vi "sv_Check for AvgParam Change [Octave].vi"(6 "averaging type":T2(ring), 7 "restart averaging (F) /reset":bool, 8 "error in (no error)":errorcluster, 9 "equal confidence level [dB]":dbl=1.0 format="%.2f", 10 "exp avg settings":T1={" mode"=enum."Fast", "time constant [ms]"=125.0} {"time constant [ms]" format="%.2f"}) -> (0 "error out":errorcluster, 2 "Param_has_changed":bool)   [LabVIEW 2017, in "SoundVib_Octave_2014 standard.lvlib"]
uses:
  <vilib>/addons/Sound and Vibration/svt_Octave/SoundVib_Octave_2014 standard.lvlib
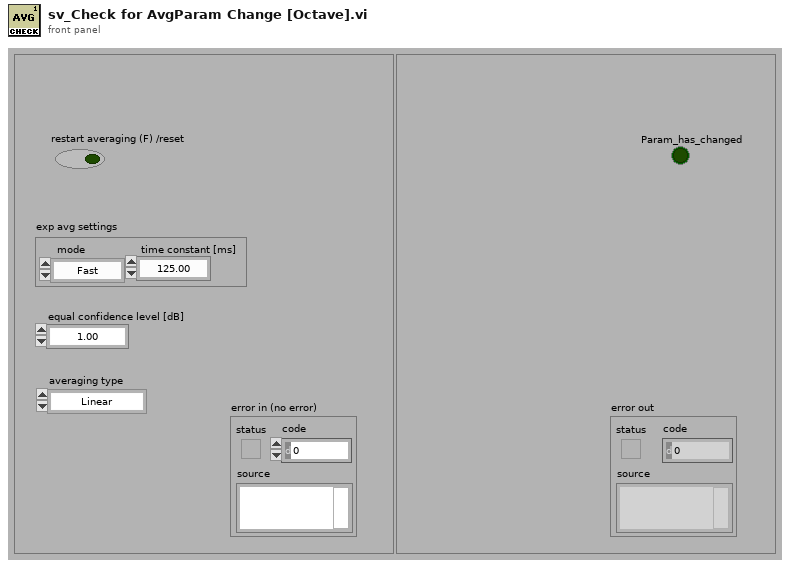
[diagram p1: front panel]
types:
  T1 = cluster{" mode":enum16{"Slow", "Fast", "Impulse", "Custom"}, "time constant [ms]":dbl}
  T2 = enum16{"Linear", "Exponential", "Equal confidence", "Peak"}
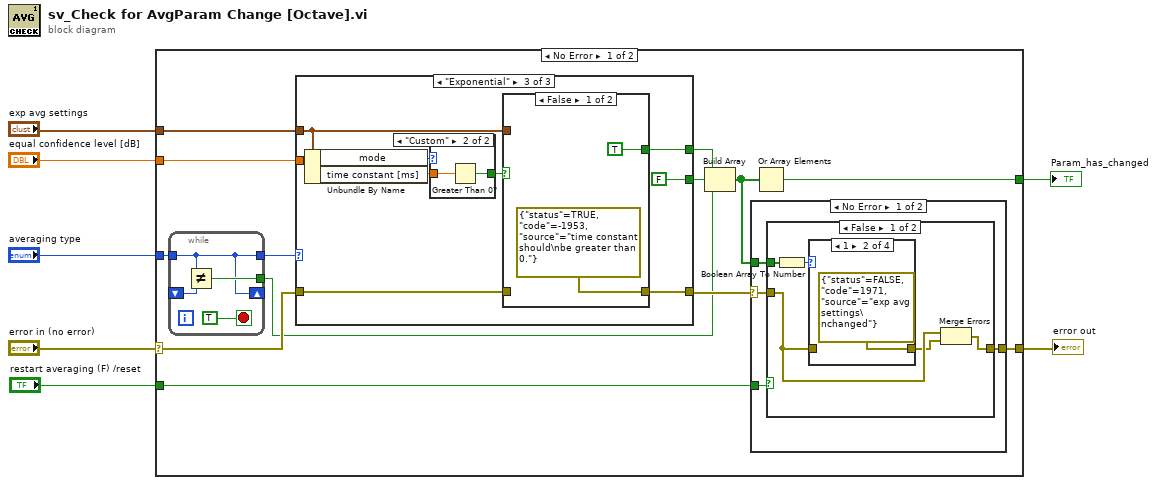
[diagram p0: block diagram]
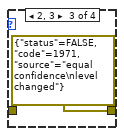
[diagram p3: hidden frame]
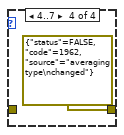
[diagram p4: hidden frame]
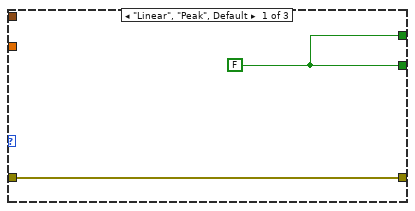
[diagram p7: hidden frame]
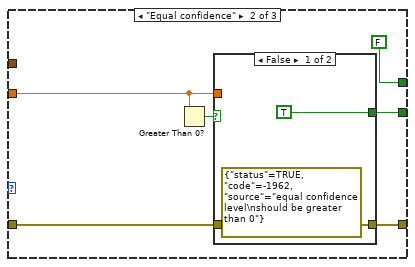
[diagram p8: hidden frame]
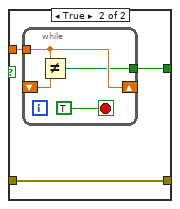
[diagram p9: hidden frame]
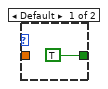
[diagram p10: hidden frame]
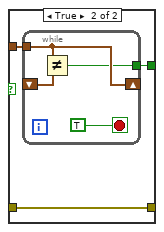
[diagram p11: hidden frame]
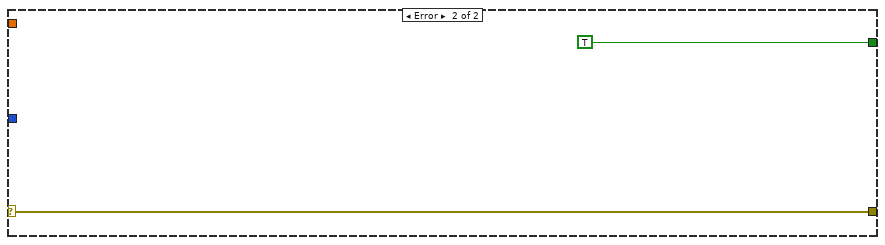
[diagram p12: hidden frame]
diagram:
  n1 = case shown="No Error" "error in (no error)" {
    selector: "error in (no error)" -> [w16 w78]
    tunnel: "exp avg settings" -> [w19 _]
    tunnel: "equal confidence level [dB]" -> [w20 _]
    tunnel: "averaging type" -> [w18 _]
    tunnel: [w9 TRUE ("status")] -> w4
    tunnel: [w14 w78] -> w2
    tunnel: "restart averaging (F) /reset" -> [w8 _]
    frame No Error {
      n2 = while {
        tunnel: [w21] -> w17
        tunnel: [w23] -> w11
        tunnel: w18 -> [w21]
        shift-left: _ -> [w24]
        shift-right: [w21] -> _
        stop <- TRUE stop-if-true
        n3 = Not Equal?(x=w21, y=w24) -> (x != y?=w23:bool)
      }
      n4 = case shown="\"Exponential\"" w17 {
        tunnel: w20 -> [_ w46 _]
        tunnel: w19 -> [_ _ w62]
        tunnel: w16 -> [w40 w45 w60]
        tunnel: [w40 w44 w59] -> w15
        tunnel: [w41 w43 FALSE] -> w12
        tunnel: [w41 FALSE w63] -> w13
        frame "Linear", "Peak", Default {
          w41 = FALSE
        }
        frame "Equal confidence" {
          n5 = Greater Than 0?(x=w46) -> (x > 0?=w47:bool)
          n6 = case shown="False" w47 {
            tunnel: w46 -> [_ w52]
            tunnel: w45 -> [_ w50]
            tunnel: [errorcluster {"status"=TRUE, "code"=-1962, "source"="equal confidence level\nshould be greater than 0"} ("error IO") w50] -> w44
            tunnel: [TRUE w51] -> w43
            frame False {
            }
            frame True {
              n7 = while {
                tunnel: [w54] -> w51
                tunnel: w52 -> [w56]
                shift-left: _ -> [w55]
                shift-right: [w56] -> _
                stop <- TRUE stop-if-true
                n8 = Not Equal?(x=w56, y=w55) -> (x != y?=w54:bool)
              }
            }
          }
        }
        frame "Exponential" {
          n9 = Unbundle By Name(w62) -> ("mode"=w57:enum16{"Slow", "Fast", "Impulse", "Custom"}, "time constant [ms]"=w58:dbl)
          n10 = case shown="\"Custom\"" w57 {
            tunnel: [TRUE w67] -> w61
            tunnel: w58 -> [_ w66]
            frame Default {
            }
            frame "Custom" {
              n11 = Greater Than 0?(x=w66) -> (x > 0?=w67:bool)
            }
          }
          n12 = case shown="False" w61 {
            tunnel: w62 -> [_ w72]
            tunnel: [TRUE w71] -> w63
            tunnel: w60 -> [_ w70]
            tunnel: [errorcluster {"status"=TRUE, "code"=-1953, "source"="time constant should\nbe greater than 0."} ("error IO") w70] -> w59
            frame False {
            }
            frame True {
              n13 = while {
                tunnel: [w74] -> w71
                tunnel: w72 -> [w76]
                shift-left: _ -> [w75]
                shift-right: [w76] -> _
                stop <- TRUE stop-if-true
                n14 = Not Equal?(x=w76, y=w75) -> (x != y?=w74:bool)
              }
            }
          }
        }
      }
      n15 = Build Array(w13, w12, w11) -> (w10:bool[])
      n16 = case shown="No Error" w15 {
        selector: w15 -> [w28 w39]
        tunnel: [w27 w39] -> w14
        tunnel: w10 -> [w26 _]
        tunnel: w8 -> [w25 _]
        frame No Error {
          n17 = case shown="False" w25 {
            tunnel: w28 -> [w31 w38]
            tunnel: [w29 w38] -> w27
            tunnel: w26 -> [w32 _]
            frame False {
              n18 = Boolean Array To Number(Boolean array=w32) -> (number=w33:u32)
              n19 = case shown="1" w33 {
                tunnel: w31 -> [w34 _ _ _]
                tunnel: [w34 errorcluster {"status"=FALSE, "code"=1971, "source"="exp avg settings\nchanged"} ("error IO") errorcluster {"status"=FALSE, "code"=1971, "source"="equal confidence\nlevel changed"} ("error IO") errorcluster {"status"=FALSE, "code"=1962, "source"="averaging type\nchanged"} ("error IO")] -> w30
                frame 0, Default {
                }
                frame 1 {
                }
                frame 2, 3 {
                }
                frame 4..7 {
                }
              }
              n20 = Merge Errors(w31, w30) -> (w29:errorcluster)
            }
            frame True {
            }
          }
        }
        frame Error {
        }
      }
      n21 = Or Array Elements(Boolean array=w10) -> (logical OR=w9:bool)
    }
    frame Error {
    }
  }
  "Param_has_changed" <- w4
  "error out" <- w2
